vi "Data to JSON string Conversion.vi"(7 "Data":variant, 8 "error in":errorcluster, 9 "SubCmd":string, 10 "Command":string, 11 "Interface":string) -> (0 "error out":errorcluster, 3 "Cmd String":string)   [LabVIEW 2024]
uses:
  Host-Control's/TCP Tx-Rx cluster.ctl
  <vilib>/addons/_JKI.lib/Serialization/JSON/JKI JSON Serialization.lvlib
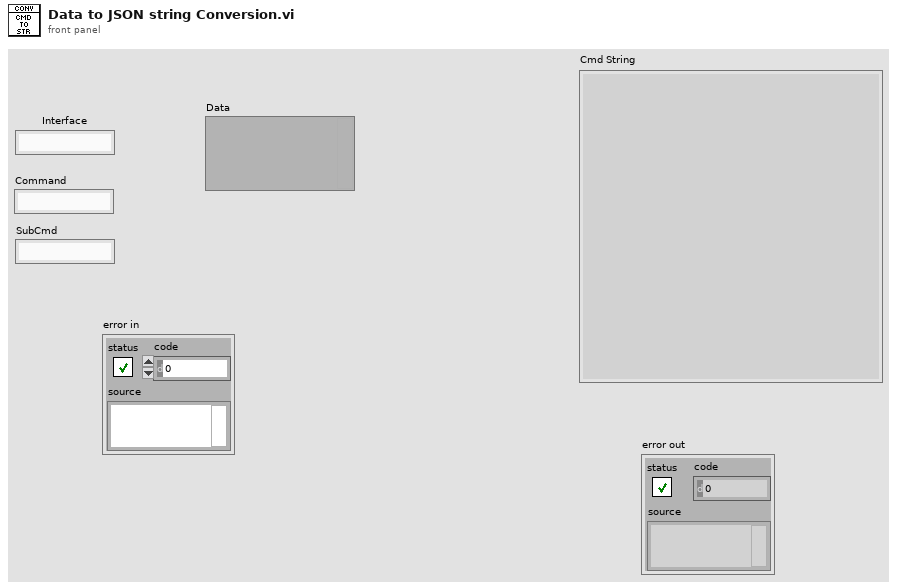
[diagram p1: front panel]
types:
  T1 = typedef "TCP Tx-Rx cluster.ctl" = cluster{"Interface":string, "Command":string, "SubCmd":string, "Data":variant}
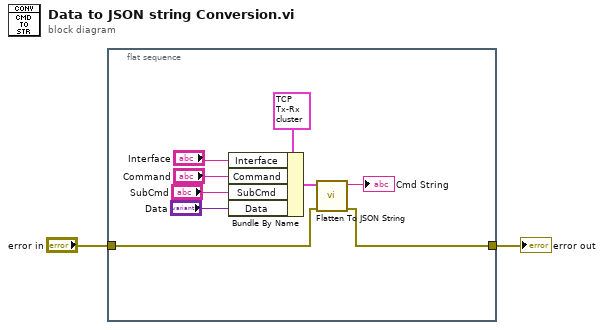
[diagram p0: block diagram]
diagram:
  n1 = flat-sequence {
    tunnel: [w3] -> w2
    tunnel: "error in" -> [w4]
    frame #0 {
      n2 = Bundle By Name(cluster=T1 {"Interface"="CPU", "Command"="CPU Info", "SubCmd"="Monitor", "Data"=variant} ("TCP Tx-Rx Cluster"), "Interface"="Interface", "Command"="Command", "SubCmd"="SubCmd", "Data"="Data") -> (w6:T1)
      n3 = call <vilib>:"Flatten To JSON String.vi"("error in"=w4, "Variant"=w6) -> ("error out"=w3:errorcluster, "JSON String"=→"Cmd String":string)  [unwired: 8 in]
    }
  }
  "error out" <- w2
